vi "下降沿.vi"(1 "Boolean Input":bool) -> (0 "Falling Edge":bool)   [LabVIEW 2015]
panel:
  out "Rising Edge":bool
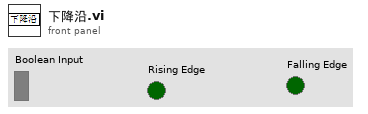
[diagram p1: front panel]
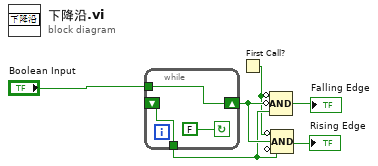
[diagram p0: block diagram]
diagram:
  n1 = while {
    tunnel: [w8] -> w5
    tunnel: "Boolean Input" -> [w9]
    shift-left: _ -> [w8]
    shift-right: [w9] -> w6
    stop <- FALSE continue-if-true
  }
  n2 = First Call?() -> (First Call?: T/F=w1:bool)
  n3 = Compound Arithmetic op=AND(invert w1, invert w6, w5) -> (→"Falling Edge":bool)
  n4 = Compound Arithmetic op=AND(invert w1, w6, invert w5) -> (→"Rising Edge":bool)
